vi "powerVsModFreq.vi"() -> ()   [LabVIEW 2016]
uses:
  <vilib>/Utility/file.llb/Write Delimited Spreadsheet (DBL).vi
panel:
  in  "number of measurements per setting":i32=10
  out "counter":i32
  out "Current freq.":dbl
  in  "file path (dialog if empty)":path
  in  "Freq step":i32=100000 format="%.2e"
  in  "End freq":dbl=20000000.0 format="%0.2e"
  in  "Start freq":dbl=100000.0 format="%0.2e"
  in  "Shuffle?":bool
  out "IDN String":string
  out "Sensor SN":string
  out "Sensor Name":string
  out "Sensor Flags":bool[](array[boolean])
  out "Readout string":string
  out "Readout value":dbl format="%^#_9e"
  in  "Timeout [ms]":i32=1000
  out "New":bool
  in  "Readout Config":string(combo)="POW"
  in  "Averaging Rate":i32=300
  out "Error log":string
  in  "Enum":enum16{"Triangle", "Sine"}(ring)
  in  "VISA resource name":refnum<visa-resource-name>="GPIB0::4::INSTR"
  in  "Serial Configuration":T1={"Baud Rate"=9600, "Parity"=0, "Data Bits"=8, "Flow Control"=4} {"Flow Control" items=["None", "XON/XOFF", "RTS/CTS", "XON/XOFF & RTS/CTS", "DTR/DSR", "XON/XOFF & DTR/DSR"]; "Data Bits" items=["7"=7, "8"=8]; "Parity" items=["None", "Odd", "Even", "Mark", "Space"]; "Baud Rate" items=["300"=300, "600"=600, "1200"=1200, "2400"=2400, "4800"=4800, "9600"=9600, "19200"=19200]}
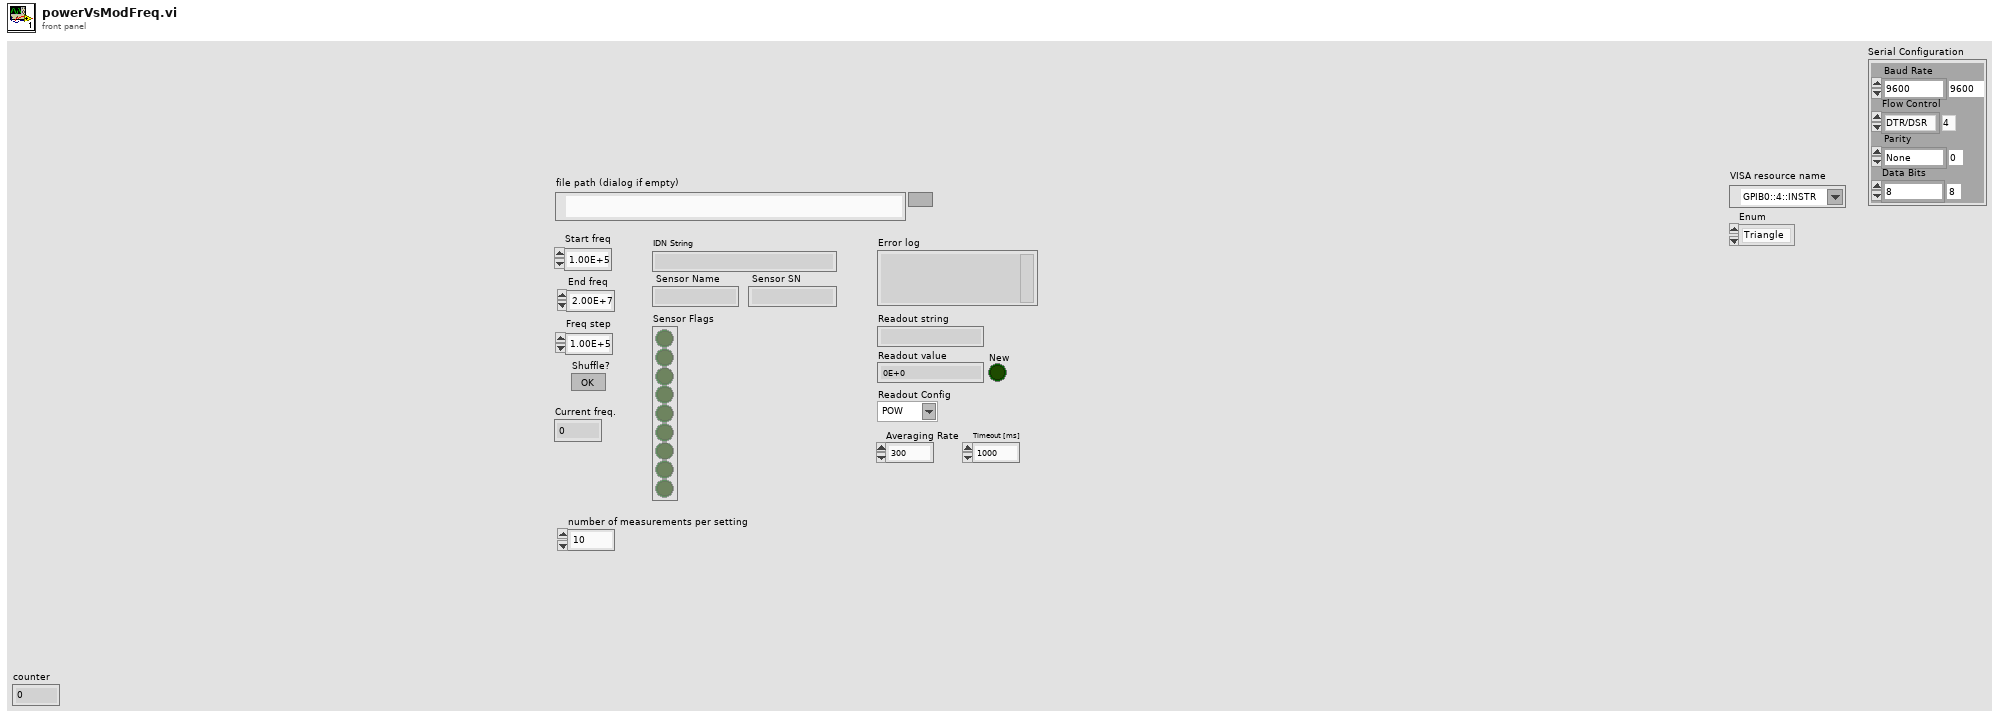
[diagram p1: front panel]
types:
  T1 = cluster{"Baud Rate":u32, "Parity":u16, "Data Bits":u16, "Flow Control":u16}
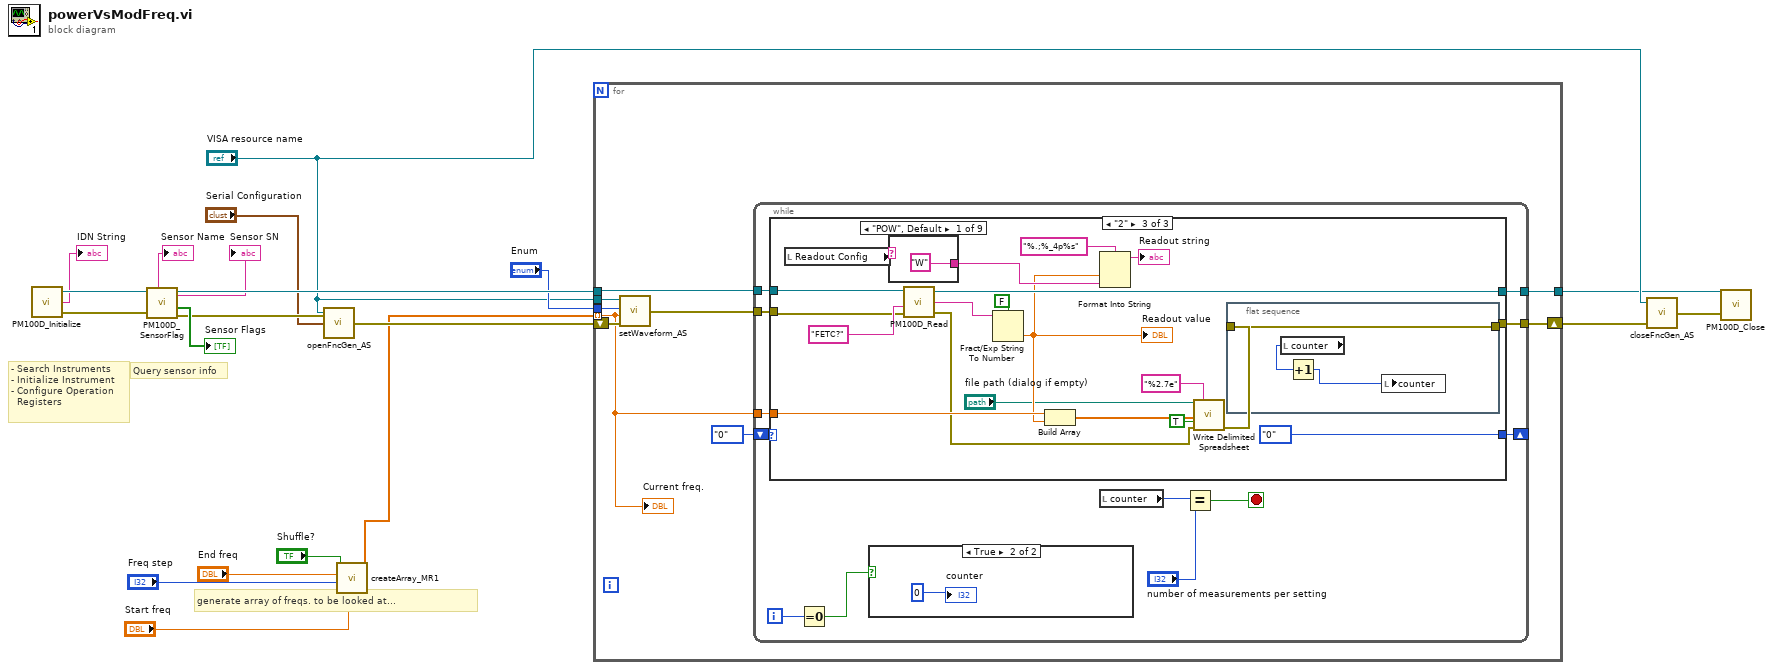
[diagram p0: block diagram]
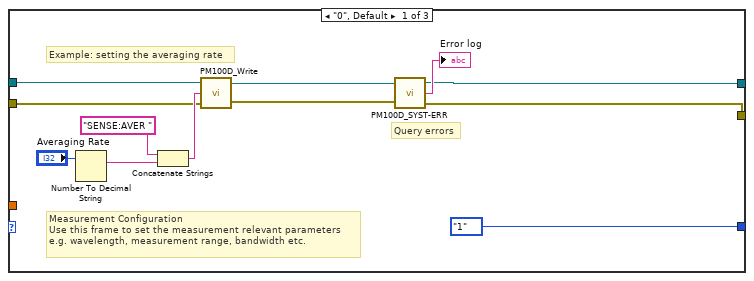
[diagram p3: hidden frame]
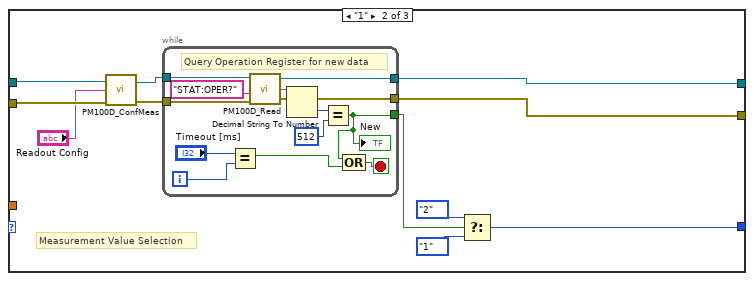
[diagram p4: hidden frame]
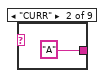
[diagram p5: hidden frame]
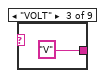
[diagram p6: hidden frame]
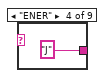
[diagram p7: hidden frame]
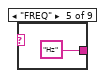
[diagram p8: hidden frame]
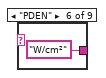
[diagram p9: hidden frame]
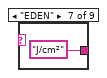
[diagram p10: hidden frame]
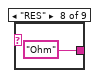
[diagram p11: hidden frame]
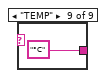
[diagram p12: hidden frame]
diagram:
  # "generate array of freqs. to be looked at..."
  # "- Search Instruments\n- Initialize Instrument\n- Configure Operation\n  Registers"
  # "Query sensor info"
  n1 = call "PM100D_Initialize.vi"() -> ("error out"=w19:errorcluster, "Instrument"=→"IDN String":string, "VISA out"=w20:refnum<visa-resource-name>)  [unwired: 2 in, 1 out]
  n2 = call "PM100D_SensorFlag.vi"("error in (no error)"=w19, "VISA in"=w20) -> ("error out"=w13:errorcluster, "flags"=→"Sensor Flags":bool[], "VISA out"=w18:refnum<visa-resource-name>, "sn"=→"Sensor SN":string, "name"=→"Sensor Name":string)  [unwired: 2 in, 3 out]
  n3 = call "openFncGen_AS.vi"("error in (no error)"=w13, "Serial Configuration"="Serial Configuration", "VISA resource name"="VISA resource name") -> ("error out"=w7:errorcluster)
  n4 = call "createArray_MR1.vi"("Start freq"="Start freq", "Freq step"="Freq step", "End freq"="End freq", "Shuffle?"="Shuffle?") -> ("Riffled {X}"=w6:dbl[])  [unwired: 7 in]
  n5 = for {
    tunnel: w18 -> [w29]
    tunnel: w6 -> [w21] mode=indexing
    tunnel: "VISA resource name" -> [w25]
    tunnel: "Enum" -> [w24]
    tunnel: [w23] -> w1
    shift-right: [w22] -> w4
    shift-left: w7 -> [w27]
    n6 = call "setWaveform_AS.vi"("error in (no error)"=w27, "Frequency (1000 Hz)"=w21, "Enum"=w24, "VISA resource name"=w25) -> ("error out"=w26:errorcluster)
    n7 = while {
      tunnel: w29 -> [w41]
      tunnel: w26 -> [w40]
      shift-right: [w38] -> _
      shift-left: enum16{"0", "1", "2"}."0" -> [w39]
      tunnel: [w37] -> w23
      tunnel: [w36] -> w22
      tunnel: w21 -> [w35]
      i -> [w31]
      stop <- w34 stop-if-true
      n8 = case shown="\"2\"" w39 {
        tunnel: w41 -> [w51 w65 w96]
        tunnel: w40 -> [w46 w64 w95]
        tunnel: [enum16{"0", "1", "2"}."1" w59 enum16{"0", "1", "2"}."0"] -> w38
        tunnel: [w44 w61 w94] -> w37
        tunnel: [w43 w60 w79] -> w36
        tunnel: w35 -> [_ _ w85]
        frame "0", Default {
          # "Query errors"
          # "Example: setting the averaging rate"
          # "Measurement Configuration\nUse this frame to set the measurement relevant parameters\ne.g. wavelength, measurement range, bandwidth etc."
          n9 = Number To Decimal String(number="Averaging Rate") -> (decimal integer string=w53:string)  [unwired: 1 in]
          n10 = Concatenate Strings("SENSE:AVER " ("string"), w53) -> (w50:string)
          n11 = call "PM100D_Write.vi"("error in (no error)"=w46, "Command"=w50, "VISA in"=w51) -> ("error out"=w47:errorcluster, "VISA out"=w49:refnum<visa-resource-name>)
          n12 = call "PM100D_SYST-ERR.vi"("error out 2"=w47, "VISA In"=w49) -> ("error out"=w43:errorcluster, "Error"=→"Error log":string, "VISA Out"=w44:refnum<visa-resource-name>)  [unwired: 1 in]
        }
        frame "1" {
          # "Measurement Value Selection"
          n13 = call "PM100D_ConfMeas.vi"("error in"=w64, "Conf:"="Readout Config", "VISA In"=w65) -> ("error out"=w62:errorcluster, "dup VISA session"=w63:refnum<visa-resource-name>)
          n14 = while {
            tunnel: w63 -> [w74]
            tunnel: w62 -> [w73]
            tunnel: [w72] -> w61
            tunnel: [w71] -> w60
            tunnel: [w66] -> w56
            i -> [w68]
            stop <- w70 stop-if-true
            # "Query Operation Register for new data"
            n15 = Equal?(x="Timeout [ms]", y=w68) -> (x = y?=w67:bool)
            n16 = call "PM100D_Read.vi"("error in (no error)"=w73, "Command"="STAT:OPER?", "VISA in"=w74) -> ("error out"=w71:errorcluster, "ReadValue"=w77:string, "VISA out"=w72:refnum<visa-resource-name>)  [unwired: 1 in]
            n17 = Decimal String To Number(string=w77) -> (number=w76:i32)  [unwired: 2 in, 1 out]
            n18 = Equal?(x=w76, y=512) -> (x = y?=w66:bool)
            "New" <- w66
            n19 = Compound Arithmetic op=OR(w66, w67) -> (w70:bool)
          }
          n20 = Select(t=enum16{"0", "1", "2"}."2", s=w56, f=enum16{"0", "1", "2"}."1") -> (s? t:f=w59:enum16{"0", "1", "2"})
        }
        frame "2" {
          n21 = local read "Readout Config"() -> (w93:string)
          n22 = case shown="\"POW\", Default" w93 {
            tunnel: ["W" "A" "V" "J" "Hz" "W/cm²" "J/cm²" "Ohm" "°C"] -> w89
            frame "POW", Default {
            }
            frame "CURR" {
            }
            frame "VOLT" {
            }
            frame "ENER" {
            }
            frame "FREQ" {
            }
            frame "PDEN" {
            }
            frame "EDEN" {
            }
            frame "RES" {
            }
            frame "TEMP" {
            }
          }
          n23 = call "PM100D_Read.vi"("error in (no error)"=w95, "Command"="FETC?", "VISA in"=w96) -> ("error out"=w81:errorcluster, "ReadValue"=w92:string, "VISA out"=w94:refnum<visa-resource-name>)  [unwired: 1 in]
          n24 = Fract/Exp String To Number(use system decimal point (T)=FALSE, string=w92) -> (number=w84:dbl)  [unwired: 2 in, 1 out]
          "Readout value" <- w84
          n25 = Build Array(w85, w84) -> (w83:dbl[])
          n26 = Format Into String(format string="%.;%_4p%s", w84, w89) -> (resulting string=→"Readout string":string)  [unwired: 2 in, 1 out]
          n27 = call-poly <vilib>:"Write Delimited Spreadsheet.vi"("file path (dialog if empty)"="file path (dialog if empty)", "format (%.3f)"="%2.7e", "1D data"=w83, "append to file? (new file:F)"=TRUE, "error in (no error)"=w81) -> ("error out"=w80:errorcluster)  [unwired: 9 in, 1 out]
          n28 = flat-sequence {
            tunnel: w80 -> [w101]
            tunnel: [w101] -> w79
            frame #0 {
              n29 = local read "counter"() -> (w100:i32)
              n30 = Increment(x=w100) -> (x+1=w99:i32)
              n31 = local write "counter"(w99) -> ()
            }
          }
        }
      }
      n32 = Equal To 0?(x=w31) -> (x = 0?=w32:bool)
      n33 = case shown="True" w32 {
        frame False {
        }
        frame True {
          "counter" <- 0 ("counter")
        }
      }
      n34 = local read "counter"() -> (w30:i32)
      n35 = Equal?(x=w30, y="number of measurements per setting") -> (x = y?=w34:bool)
    }
    "Current freq." <- w21
  }
  n36 = call "closeFncGen_AS.vi"("error in (no error)"=w4, "VISA resource name"="VISA resource name") -> ("error out"=w2:errorcluster)  [unwired: 1 in]
  n37 = call "PM100D_Close.vi"("error in (no error)"=w2, "VISA resource name"=w1) -> ()  [unwired: 2 in]
